vi "pause.vi"() -> (0 "User's choice":string)   [LabVIEW 2025]
panel:
  in  "Retry":bool
  in  "Quit":bool
  in  "Continue":bool
  out "Paused, replay?":string="Paused.\nResume play?"
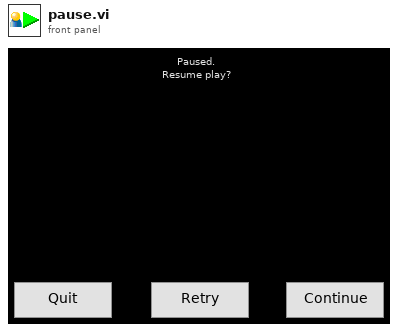
[diagram p1: front panel]
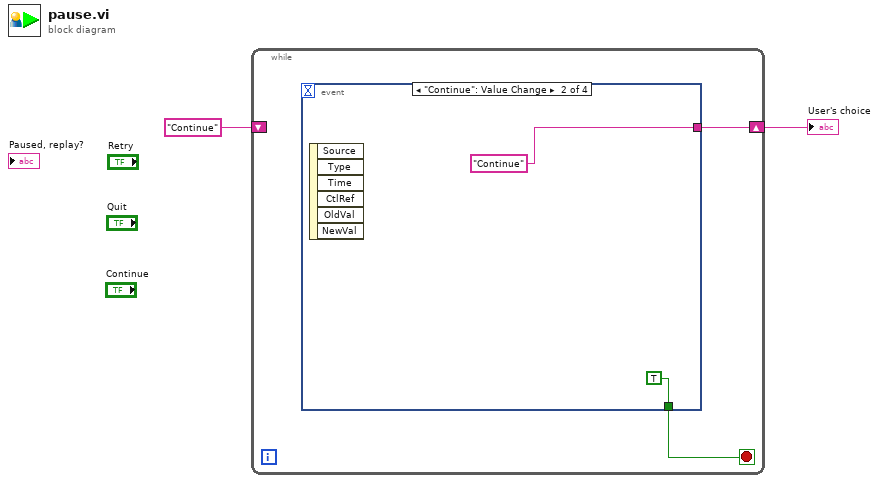
[diagram p0: block diagram]
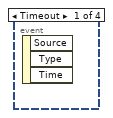
[diagram p2: hidden frame]
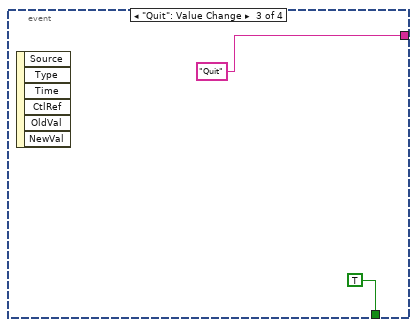
[diagram p3: hidden frame]
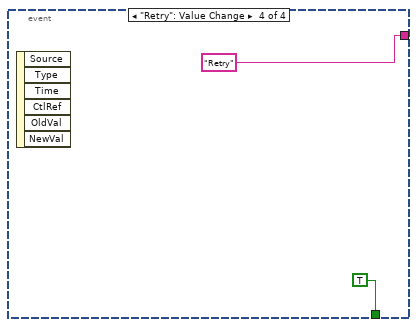
[diagram p4: hidden frame]
diagram:
  n1 = while {
    shift-right: [w3] -> w1
    shift-left: "Continue" -> [_]
    stop <- w4 stop-if-true
    n2 = event shown="[1] \"Continue\": Value Change" {
      selector: _ -> [_ _ _ _]
      dyn-events: _ -> [_ _ _ _]
      timeout: _ -> [_ _ _ _]
      tunnel: [_ TRUE TRUE TRUE] -> w4
      tunnel: [_ "Continue" "Quit" "Retry"] -> w3
      event Timeout {
        n3 = event-data() -> ()  [unwired: 1 in, 3 out]
      }
      event "Continue": Value Change {
        n4 = event-data() -> ()  [unwired: 1 in, 6 out]
      }
      event "Quit": Value Change {
        n5 = event-data() -> ()  [unwired: 1 in, 6 out]
      }
      event "Retry": Value Change {
        n6 = event-data() -> ()  [unwired: 1 in, 6 out]
      }
    }
  }
  "User's choice" <- w1
